vi "Get Path Main.vi"(8 "error in (no error)":errorcluster) -> (0 "error out":errorcluster, 3 "All Path":T1)   [LabVIEW 2017]
uses:
  Controls/Get Path - All Path Control.ctl
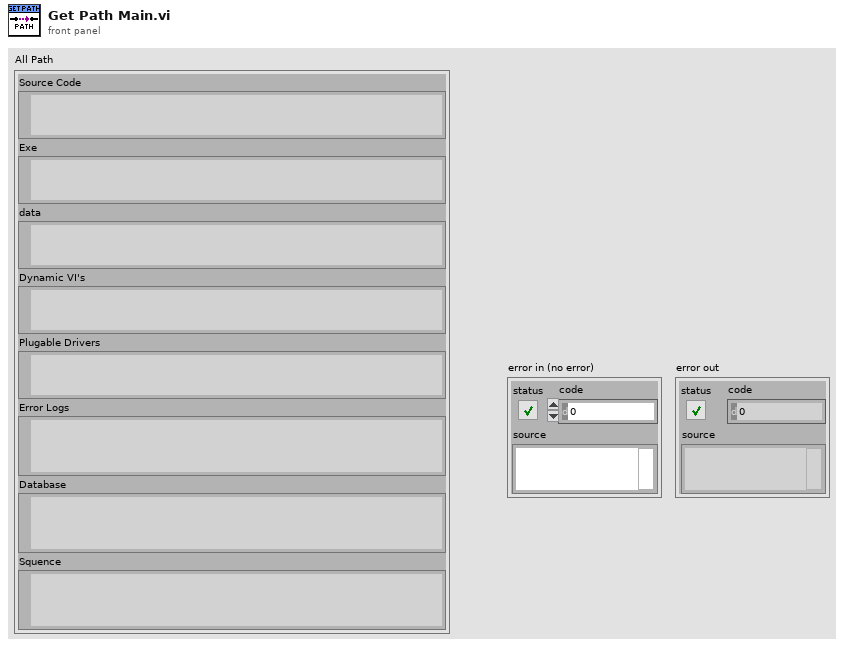
[diagram p1: front panel]
types:
  T1 = typedef "Get Path - All Path Control.ctl" = cluster{"Source Code":path, "Exe":path, "data":path, "Dynamic VI's":path, "Plugable Drivers":path, "Error Logs":path, "Database":path, "Squence":path}
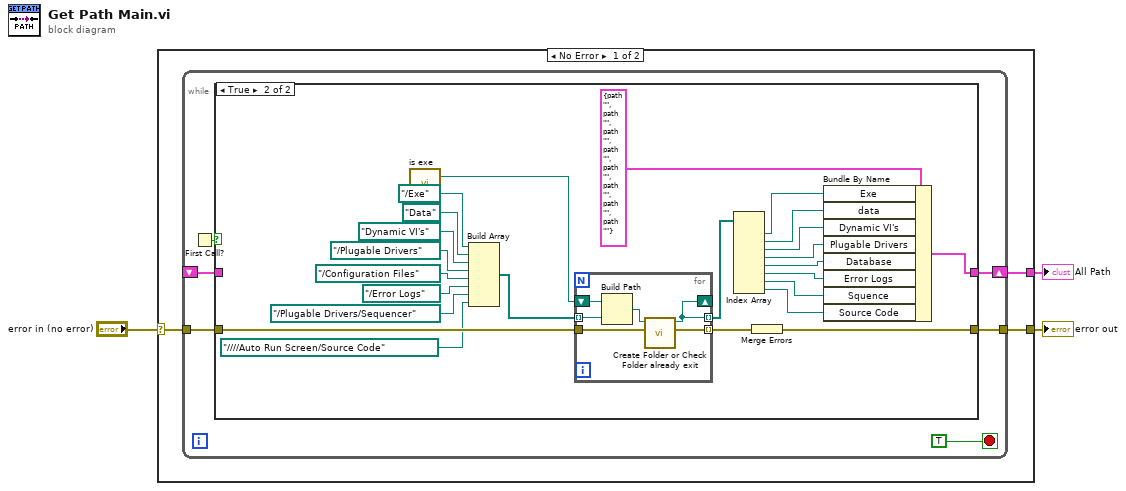
[diagram p0: block diagram]
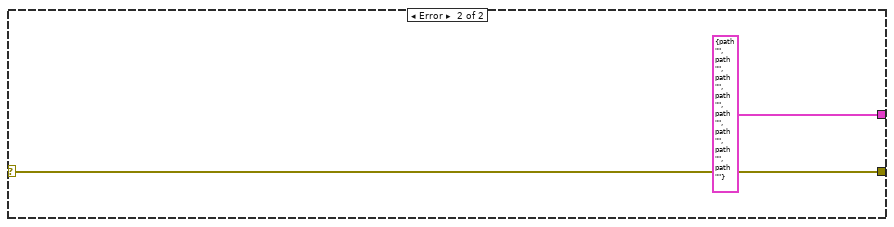
[diagram p3: hidden frame]
diagram:
  n1 = case shown="No Error" "error in (no error)" {
    selector: "error in (no error)" -> [w5 w46]
    tunnel: [w6 w46] -> w2
    tunnel: [w4 T1 {"Source Code"=path "", "Exe"=path "", "data"=path "", "Dynamic VI's"=path "", "Plugable Drivers"=path "", "Error Logs"=path "", "Database"=path "", "Squence"=path ""} ("All Path")] -> w1
    frame No Error {
      n2 = while {
        tunnel: [w10] -> w6
        tunnel: w5 -> [w9]
        shift-right: [w8] -> w4
        shift-left: _ -> [w7]
        stop <- TRUE stop-if-true
        n3 = First Call?() -> (First Call?: T/F=w11:bool)
        n4 = case shown="True" w11 {
          tunnel: [w14 w35] -> w10
          tunnel: w9 -> [w14 w23]
          tunnel: [w13 w37] -> w8
          tunnel: w7 -> [w13 _]
          frame False {
          }
          frame True {
            n5 = call "is exe.vi"() -> ("Path"=w22:path)  [unwired: 3 in]
            n6 = Build Array(path "../Exe" ("Path"), path "Data" ("Path"), path "Dynamic VI's" ("Path"), path "../Plugable Drivers" ("Path"), path "../Configuration Files" ("Path"), path "../Error Logs" ("Path"), path "../Plugable Drivers/Sequencer" ("element"), path "../../../../Auto Run Screen/Source Code" ("Path")) -> (w34:path[])
            n7 = for {
              tunnel: w34 -> [w41] mode=indexing
              tunnel: [w39] -> w30 mode=indexing
              tunnel: w23 -> [w43]
              tunnel: [w44] -> w36 mode=indexing
              shift-right: [w39] -> _
              shift-left: w22 -> [w42]
              n8 = Build Path(base path=w42, name or relative path=w41) -> (appended path=w40:path)
              n9 = call "Create Folder or Check Folder already exit.vi"("error in (no error)"=w43, "Path In"=w40) -> ("error out"=w44:errorcluster, "Path Out"=w39:path)  [unwired: 4 in]
            }
            n10 = Index Array(array=w30) -> (element #1=w29:path, element #2=w33:path, element #3=w32:path, element #4=w31:path, element #5=w19:path, element #6=w18:path, element #7=w16:path, element #8=w15:path)  [unwired: 8 in]
            n11 = Merge Errors(w36) -> (w35:errorcluster)
            n12 = Bundle By Name(cluster=T1 {"Source Code"=path "", "Exe"=path "", "data"=path "", "Dynamic VI's"=path "", "Plugable Drivers"=path "", "Error Logs"=path "", "Database"=path "", "Squence"=path ""} ("All Path"), "Exe"=w29, "data"=w33, "Dynamic VI's"=w32, "Plugable Drivers"=w31, "Database"=w19, "Error Logs"=w18, "Squence"=w16, "Source Code"=w15) -> (w37:T1)
          }
        }
      }
    }
    frame Error {
    }
  }
  "error out" <- w2
  "All Path" <- w1
